vi "S2C_XML_UpdateElement.vi"(8 "Error In":errorcluster, 10 "Value":string, 11 "Xpath":string) -> (0 "Error Out":errorcluster)   [LabVIEW 2015]
uses:
  S2C_XML_Globals.vi
  <vilib>/xml/Close Reference(Node).vi
  <resource>/objmgr/DOMUserDefRef.rc
  <vilib>/xml/NI_XML.lvlib
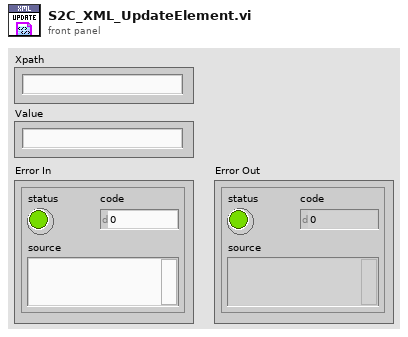
[diagram p1: front panel]
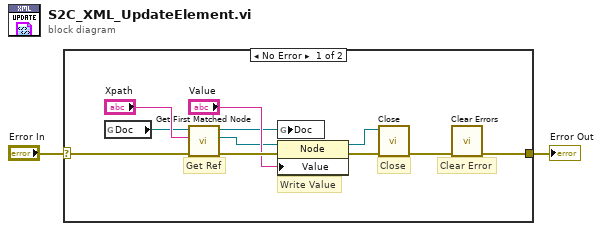
[diagram p0: block diagram]
diagram:
  n1 = case shown="No Error" "Error In" {
    selector: "Error In" -> [w9 w14]
    tunnel: [w5 w14] -> w2
    frame No Error {
      # "Clear Error"
      # "Write Value"
      # "Close"
      # "Get Ref"
      n2 = global read "S2C_XML_Globals.vi" "Doc"() -> (w12:refnum<k20>)
      n3 = call <vilib>:"Get First Matched Node.vi"("error in (no error)"=w9, "XPath expression"="Xpath", "node in"=w12) -> ("error out"=w11:errorcluster, "node result"=w8:refnum<k20>, "node out"=w7:refnum<k20>)  [unwired: 6 in]
      n4 = global write "S2C_XML_Globals.vi" "Doc"(w7) -> ()
      n5 = property class="Node"(reference=w8, error in=w11, "Value"="Value") -> (reference out=w3:refnum<k20>, error out=w4:errorcluster)
      n6 = call-poly <vilib>:"Close.vi"("error in (no error)"=w4, "node"=w3) -> ("error out"=w6:errorcluster)  [unwired: 7 in]
      n7 = call <vilib>:"Clear Errors.vi"("error in (no error)"=w6) -> ("error out"=w5:errorcluster)  [unwired: 5 in, 1 out]
    }
    frame Error {
    }
  }
  "Error Out" <- w2
